vi "oax_AI Config (DAQmx).vi"(0 "master":T1={"DSA Device"="", "Channels"={"enable ch0"=TRUE, "enable ch1"=TRUE, "enable ch2"=FALSE, "enable ch3"=FALSE, "enable ch4"=FALSE, "enable ch5"=FALSE, "enable ch6"=FALSE, "enable ch7"=FALSE}, "Channel Names"={"ch0 string"="Tachometer", "ch1 string"="Acc1", "ch2 string"="", "ch3 string"="", "ch4 string"="", "ch5 string"="", "ch6 string"="", "ch7 string"=""}, "Coupling"={"coupling ch0"=FALSE, "coupling ch1"=FALSE, "coupling ch2"=FALSE, "coupling ch3"=FALSE, "coupling ch4"=FALSE, "coupling ch5"=FALSE, "coupling ch6"=FALSE, "coupling ch7"=FALSE}, "IEPE"={"ICP ch0"=TRUE, "ICP ch0"=FALSE, "ICP ch0"=FALSE, "ICP ch0"=FALSE, "ICP ch0"=FALSE, "ICP ch0"=FALSE, "ICP ch0"=FALSE, "ICP ch0"=FALSE}, "Ch. Sensitivity\n[mV/EU]"={"ch0 sensitivity"=1000.0, "ch1 sensitivity"=1000.0, "ch2 sensitivity"=1000.0, "ch3 sensitivity"=1000.0, "ch4 sensitivity"=1000.0, "ch5 sensitivity"=1000.0, "ch6 sensitivity"=1000.0, "ch7 sensitivity"=1000.0}, "Engineering\nUnits"={"Engineering\nUnits"=1000, "Engineering\nUnits"=100, "Engineering\nUnits"=1000, "Engineering\nUnits"=1000, "Engineering\nUnits"=1000, "Engineering\nUnits"=1000, "Engineering\nUnits"=1000, "Engineering\nUnits"=1000}, "Custom\nLabel"={"Custom Label"="", "Custom Label"="", "Custom Label"="", "Custom Label"="", "Custom Label"="", "Custom Label"="", "Custom Label"="", "Custom Label"=""}, "dB reference\n[EU]"={"dB reference [EU]"=1.0, "dB reference [EU]"=1.0, "dB reference [EU]"=1.0, "dB reference [EU]"=1.0, "dB reference [EU]"=1.0, "dB reference [EU]"=1.0, "dB reference [EU]"=1.0, "dB reference [EU]"=1.0}, "pregain\n[dB]"={"pregain [dB]"=1.0, "pregain [dB]"=1.0, "pregain [dB]"=1.0, "pregain [dB]"=1.0, "pregain [dB]"=1.0, "pregain [dB]"=1.0, "pregain [dB]"=1.0, "pregain [dB]"=1.0}, "Weighting\nFilter"={"Weighting Filter"=1, "Weighting Filter"=1, "Weighting Filter"=1, "Weighting Filter"=1, "Weighting Filter"=1, "Weighting Filter"=1, "Weighting Filter"=1, "Weighting Filter"=1}, "max value"=5.0, "min value"=5.0, "enable EAR?"=FALSE} {"min value" format="%0.2f"; "max value" format="%0.2f"; "Weighting\nFilter"."Weighting Filter" items=["Linear", "A-weighting", "B-weighting", "C-weighting", "ITU-R 468-4", "Dolby", "CCITT", "C-message"]; "Weighting\nFilter"."Weighting Filter" items=["Linear", "A-weighting", "B-weighting", "C-weighting", "ITU-R 468-4", "Dolby", "CCITT", "C-message"]; "Weighting\nFilter"."Weighting Filter" items=["Linear", "A-weighting", "B-weighting", "C-weighting", "ITU-R 468-4", "Dolby", "CCITT", "C-message"]; "Weighting\nFilter"."Weighting Filter" items=["Linear", "A-weighting", "B-weighting", "C-weighting", "ITU-R 468-4", "Dolby", "CCITT", "C-message"]; "Weighting\nFilter"."Weighting Filter" items=["Linear", "A-weighting", "B-weighting", "C-weighting", "ITU-R 468-4", "Dolby", "CCITT", "C-message"]; "Weighting\nFilter"."Weighting Filter" items=["Linear", "A-weighting", "B-weighting", "C-weighting", "ITU-R 468-4", "Dolby", "CCITT", "C-message"]; "Weighting\nFilter"."Weighting Filter" items=["Linear", "A-weighting", "B-weighting", "C-weighting", "ITU-R 468-4", "Dolby", "CCITT", "C-message"]; "Weighting\nFilter"."Weighting Filter" items=["Linear", "A-weighting", "B-weighting", "C-weighting", "ITU-R 468-4", "Dolby", "CCITT", "C-message"]; "pregain\n[dB]"."pregain [dB]" format="%.2f"; "pregain\n[dB]"."pregain [dB]" format="%.2f"; "pregain\n[dB]"."pregain [dB]" format="%.2f"; "pregain\n[dB]"."pregain [dB]" format="%.2f"; "pregain\n[dB]"."pregain [dB]" format="%.2f"; "pregain\n[dB]"."pregain [dB]" format="%.2f"; "pregain\n[dB]"."pregain [dB]" format="%.2f"; "pregain\n[dB]"."pregain [dB]" format="%.2f"; "dB reference\n[EU]"."dB reference [EU]" format="%^.1e"; "dB reference\n[EU]"."dB reference [EU]" format="%^.1e"; "dB reference\n[EU]"."dB reference [EU]" format="%^.1e"; "dB reference\n[EU]"."dB reference [EU]" format="%^.1e"; "dB reference\n[EU]"."dB reference [EU]" format="%^.1e"; "dB reference\n[EU]"."dB reference [EU]" format="%^.1e"; "dB reference\n[EU]"."dB reference [EU]" format="%^.1e"; "dB reference\n[EU]"."dB reference [EU]" format="%^.1e"; "Engineering\nUnits"."Engineering\nUnits" items=["custom..."=0, "V"=1, "A"=21, "Pa"=2, "N"=20, "g"=3, "m/s^2"=4, "m/s"=5, "m"=6, "mm/s"=12, "mm"=13, "microns/s"=14, "microns"=15, "in/s^2"=7, "in/s"=8, "in"=9, "mils/s"=10, "mils"=11, "rad/s^2"=16, "rad/s"=17, "rad"=18, "strain"=19]; "Engineering\nUnits"."Engineering\nUnits" items=["custom..."=0, "V"=1, "A"=21, "Pa"=2, "N"=20, "g"=3, "m/s^2"=4, "m/s"=5, "m"=6, "mm/s"=12, "mm"=13, "microns/s"=14, "microns"=15, "in/s^2"=7, "in/s"=8, "in"=9, "mils/s"=10, "mils"=11, "rad/s^2"=16, "rad/s"=17, "rad"=18, "strain"=19]; "Engineering\nUnits"."Engineering\nUnits" items=["custom..."=0, "V"=1, "A"=21, "Pa"=2, "N"=20, "g"=3, "m/s^2"=4, "m/s"=5, "m"=6, "mm/s"=12, "mm"=13, "microns/s"=14, "microns"=15, "in/s^2"=7, "in/s"=8, "in"=9, "mils/s"=10, "mils"=11, "rad/s^2"=16, "rad/s"=17, "rad"=18, "strain"=19]; "Engineering\nUnits"."Engineering\nUnits" items=["custom..."=0, "V"=1, "A"=21, "Pa"=2, "N"=20, "g"=3, "m/s^2"=4, "m/s"=5, "m"=6, "mm/s"=12, "mm"=13, "microns/s"=14, "microns"=15, "in/s^2"=7, "in/s"=8, "in"=9, "mils/s"=10, "mils"=11, "rad/s^2"=16, "rad/s"=17, "rad"=18, "strain"=19]; "Engineering\nUnits"."Engineering\nUnits" items=["custom..."=0, "V"=1, "A"=21, "Pa"=2, "N"=20, "g"=3, "m/s^2"=4, "m/s"=5, "m"=6, "mm/s"=12, "mm"=13, "microns/s"=14, "microns"=15, "in/s^2"=7, "in/s"=8, "in"=9, "mils/s"=10, "mils"=11, "rad/s^2"=16, "rad/s"=17, "rad"=18, "strain"=19]; "Engineering\nUnits"."Engineering\nUnits" items=["custom..."=0, "V"=1, "A"=21, "Pa"=2, "N"=20, "g"=3, "m/s^2"=4, "m/s"=5, "m"=6, "mm/s"=12, "mm"=13, "microns/s"=14, "microns"=15, "in/s^2"=7, "in/s"=8, "in"=9, "mils/s"=10, "mils"=11, "rad/s^2"=16, "rad/s"=17, "rad"=18, "strain"=19]; "Engineering\nUnits"."Engineering\nUnits" items=["custom..."=0, "V"=1, "A"=21, "Pa"=2, "N"=20, "g"=3, "m/s^2"=4, "m/s"=5, "m"=6, "mm/s"=12, "mm"=13, "microns/s"=14, "microns"=15, "in/s^2"=7, "in/s"=8, "in"=9, "mils/s"=10, "mils"=11, "rad/s^2"=16, "rad/s"=17, "rad"=18, "strain"=19]; "Engineering\nUnits"."Engineering\nUnits" items=["custom..."=0, "V"=1, "A"=21, "Pa"=2, "N"=20, "g"=3, "m/s^2"=4, "m/s"=5, "m"=6, "mm/s"=12, "mm"=13, "microns/s"=14, "microns"=15, "in/s^2"=7, "in/s"=8, "in"=9, "mils/s"=10, "mils"=11, "rad/s^2"=16, "rad/s"=17, "rad"=18, "strain"=19]; "Ch. Sensitivity\n[mV/EU]"."ch7 sensitivity" format="%.2f"; "Ch. Sensitivity\n[mV/EU]"."ch6 sensitivity" format="%.2f"; "Ch. Sensitivity\n[mV/EU]"."ch5 sensitivity" format="%.2f"; "Ch. Sensitivity\n[mV/EU]"."ch4 sensitivity" format="%.2f"; "Ch. Sensitivity\n[mV/EU]"."ch3 sensitivity" format="%.2f"; "Ch. Sensitivity\n[mV/EU]"."ch2 sensitivity" format="%.2f"; "Ch. Sensitivity\n[mV/EU]"."ch1 sensitivity" format="%.2f"; "Ch. Sensitivity\n[mV/EU]"."ch0 sensitivity" format="%.2f"}, 5 "buffer size":u32=10000, 11 "error in (no error)":errorcluster) -> (4 "task out":refnum<k21>, 15 "error out":errorcluster)   [LabVIEW 2017]
doc: "Reset devices and creates a DAQmx AI Voltage task, configure IEPE excitation, and input coupling."
uses:
  <vilib>/addons/Sound and Vibration/Order Analysis/Example Support/sub VIs/OAXML_Analog Channel Config (DAQmx).ctl
  <resource>/objmgr/daqmx.rc
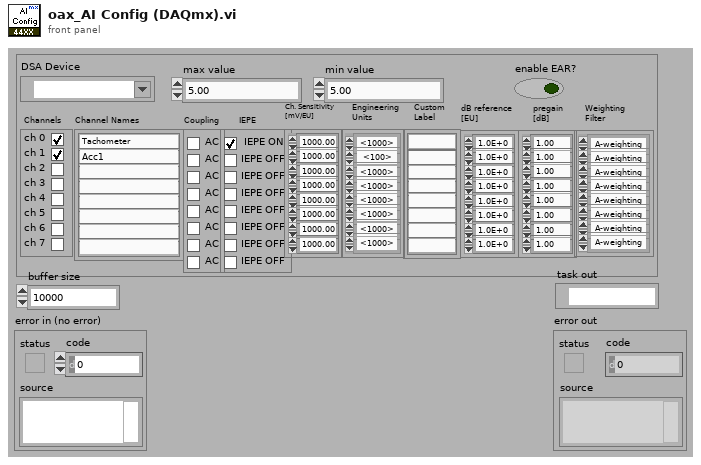
[diagram p1: front panel]
types:
  T1 = typedef "OAXML_Analog Channel Config (DAQmx).ctl" = cluster{"DSA Device":tag, "Channels":cluster{"enable ch0":bool, "enable ch1":bool, "enable ch2":bool, "enable ch3":bool, "enable ch4":bool, "enable ch5":bool, "enable ch6":bool, "enable ch7":bool}, "Channel Names":cluster{"ch0 string":string, "ch1 string":string, "ch2 string":string, "ch3 string":string, "ch4 string":string, "ch5 string":string, "ch6 string":string, "ch7 string":string}, "Coupling":cluster{"coupling ch0":bool, "coupling ch1":bool, "coupling ch2":bool, "coupling ch3":bool, "coupling ch4":bool, "coupling ch5":bool, "coupling ch6":bool, "coupling ch7":bool}, "IEPE":cluster{"ICP ch0":bool, "ICP ch0":bool, "ICP ch0":bool, "ICP ch0":bool, "ICP ch0":bool, "ICP ch0":bool, "ICP ch0":bool, "ICP ch0":bool}, "Ch. Sensitivity\n[mV/EU]":cluster{"ch0 sensitivity":dbl, "ch1 sensitivity":dbl, "ch2 sensitivity":dbl, "ch3 sensitivity":dbl, "ch4 sensitivity":dbl, "ch5 sensitivity":dbl, "ch6 sensitivity":dbl, "ch7 sensitivity":dbl}, "Engineering\nUnits":cluster{"Engineering\nUnits":u16, "Engineering\nUnits":u16, "Engineering\nUnits":u16, "Engineering\nUnits":u16, "Engineering\nUnits":u16, "Engineering\nUnits":u16, "Engineering\nUnits":u16, "Engineering\nUnits":u16}, "Custom\nLabel":cluster{"Custom Label":string, "Custom Label":string, "Custom Label":string, "Custom Label":string, "Custom Label":string, "Custom Label":string, "Custom Label":string, "Custom Label":string}, "dB reference\n[EU]":cluster{"dB reference [EU]":dbl, "dB reference [EU]":dbl, "dB reference [EU]":dbl, "dB reference [EU]":dbl, "dB reference [EU]":dbl, "dB reference [EU]":dbl, "dB reference [EU]":dbl, "dB reference [EU]":dbl}, "pregain\n[dB]":cluster{"pregain [dB]":dbl, "pregain [dB]":dbl, "pregain [dB]":dbl, "pregain [dB]":dbl, "pregain [dB]":dbl, "pregain [dB]":dbl, "pregain [dB]":dbl, "pregain [dB]":dbl}, "Weighting\nFilter":cluster{"Weighting Filter":u16, "Weighting Filter":u16, "Weighting Filter":u16, "Weighting Filter":u16, "Weighting Filter":u16, "Weighting Filter":u16, "Weighting Filter":u16, "Weighting Filter":u16}, "max value":dbl, "min value":dbl, "enable EAR?":bool}
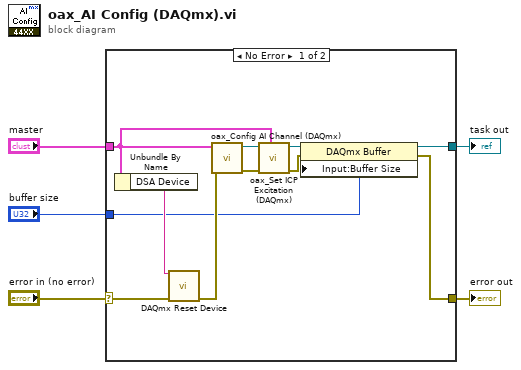
[diagram p0: block diagram]
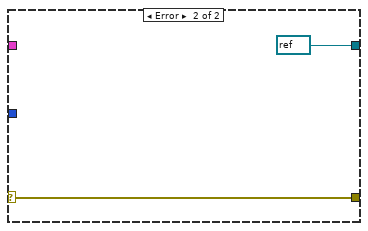
[diagram p2: hidden frame]
diagram:
  n1 = case shown="No Error" "error in (no error)" {
    selector: "error in (no error)" -> [w14 w18]
    tunnel: [w7 w18] -> w4
    tunnel: "master" -> [w12 _]
    tunnel: [w9 refnum<k21> refnum ("task out")] -> w2
    tunnel: "buffer size" -> [w6 _]
    frame No Error {
      n2 = Unbundle By Name(w12) -> ("DSA Device"=w11:tag)
      n3 = call <vilib>:"DAQmx Reset Device.vi"("device in"=w11, "error in"=w14) -> ("error out"=w13:errorcluster)  [unwired: 13 in]
      n4 = call <vilib>:"oax_Config AI Channel (DAQmx).vi"("error in (no error)"=w13, "master"=w12) -> ("error out"=w16:errorcluster, "task out"=w15:refnum<k21>)  [unwired: 8 in]
      n5 = call <vilib>:"oax_Set ICP Excitation (DAQmx).vi"("master"=w12, "error in (no error)"=w16, "task in"=w15) -> ("error out"=w8:errorcluster, "task out"=w10:refnum<k21>)  [unwired: 7 in]
      n6 = property class="DAQmx Buffer"(reference=w10, error in=w8, "Input:Buffer Size"=w6) -> (reference out=w9:refnum<k21>, error out=w7:errorcluster)
    }
    frame Error {
    }
  }
  "error out" <- w4
  "task out" <- w2
